vi "niveles.vi"(6 "Nivel cargar":dbl, 7 "Nivel step":dbl, 8 "Nivel 1 caja":dbl, 9 "Nivel 2 cajas":dbl, 10 "Nivel 3 cajas":dbl, 11 "Nivel techo":dbl) -> (2 "output cluster":T1)   [LabVIEW 2014]
panel:
  in  "Niveles elevador":T1
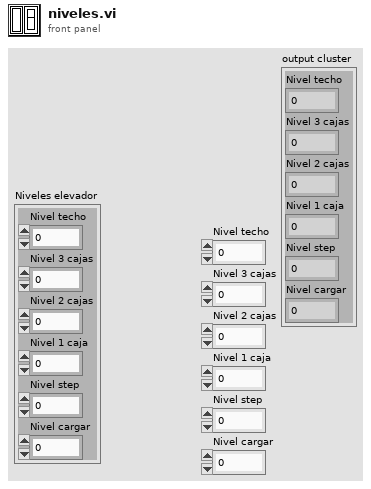
[diagram p1: front panel]
types:
  T1 = cluster{"Nivel techo":dbl, "Nivel 3 cajas":dbl, "Nivel 2 cajas":dbl, "Nivel 1 caja":dbl, "Nivel step":dbl, "Nivel cargar":dbl}
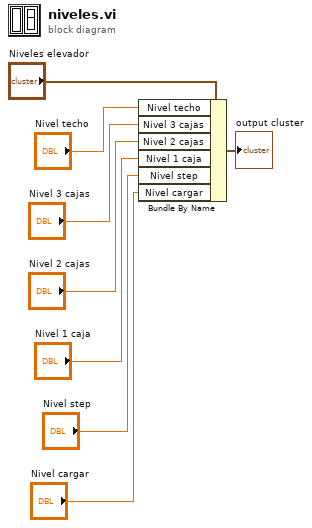
[diagram p0: block diagram]
diagram:
  n1 = Bundle By Name(cluster="Niveles elevador", "Nivel techo"="Nivel techo", "Nivel 3 cajas"="Nivel 3 cajas", "Nivel 2 cajas"="Nivel 2 cajas", "Nivel 1 caja"="Nivel 1 caja", "Nivel step"="Nivel step", "Nivel cargar"="Nivel cargar") -> (→"output cluster":T1)
